vi "Interframe_template-matched-tempbox_displacements_Checked_VI.vi"() -> ()   [LabVIEW 2012]
uses:
  <vilib>/Utility/file.llb/Write To Spreadsheet File (DBL).vi
  <vilib>/imath/engines/lvmath2/RunTimeEngine/NodeEndStatement/NIMS_NodeEndStatement_Output.vi
  <instcachedir>/0/NIMS_NodeEndStatement_Output_53EC0D466D134D7ABD903AC30B43404B.lvgen/NIMS_NodeEndStatement_Output_53EC0D466D134D7ABD903AC30B43404B_001.vi
  <instcachedir>/0/NIMS_NodeEndStatement_Output_53EC0D466D134D7ABD903AC30B43404B.lvgen/NIMS_NodeEndStatement_Output_53EC0D466D134D7ABD903AC30B43404B_005.vi
  <vilib>/imath/engines/lvmath2/RunTimeEngine/ErrorHandling/NIMS_Finalize Error.vi
panel:
  out "Frame\nDelta_X\nDelta_Z":dbl[][](array[numeric])
  out "Matched TempBox (z,x): ROI-Frame_of_Reference":i32[][](array[numeric])
  out "Min_SAD":u32[](array[numeric])
  out "Delta_Z (TempBox-Template)":dbl[](array[numeric])
  out "Delta_X (TempBox-Template)":dbl[](array[numeric])
  in  "ROI in\n2nd frame\n    s_x":dbl=623.0
  in  "ROI in\n2nd frame\n    e_x":dbl=727.0
  in  "ROI in\n2nd frame\n    s_z":dbl=272.0
  in  "ROI in\n2nd frame\n    e_z":dbl=301.0
  out "SAD":u32[][](array[numeric])
  out "SAD_1Darray":u32[](array[numeric])
  out "Frames":T1(plugin-control)
  out "Template in 1st frame of every iteration":u8[][](array[numeric])
  in  "Template \n      in\n1st frame\n     s_x":dbl=658.0
  in  "Template \n      in \n1st frame\n    s_z":dbl=282.0
  in  "Template \n      in \n1st frame\n    e_x":dbl=692.0
  in  "Template \n      in \n1st frame\n    e_z":dbl=291.0
  in  "?":bool
  in  "1st frame":dbl=153.0
  in  "Last frame":dbl=154.0
  out "framesPerSecond":u32
  out "Image Type":T2 items=["Grayscale (U8)", "Grayscale (I16)", "Grayscale (SGL)", "Complex (CSG)", "RGB (U32)", "HSL (U32)", "RGB (U64)"]
  out "Number of Frames":u32
  in  "Path":path=path "C:/Users/admin/Desktop/lohit/pat3.avi"
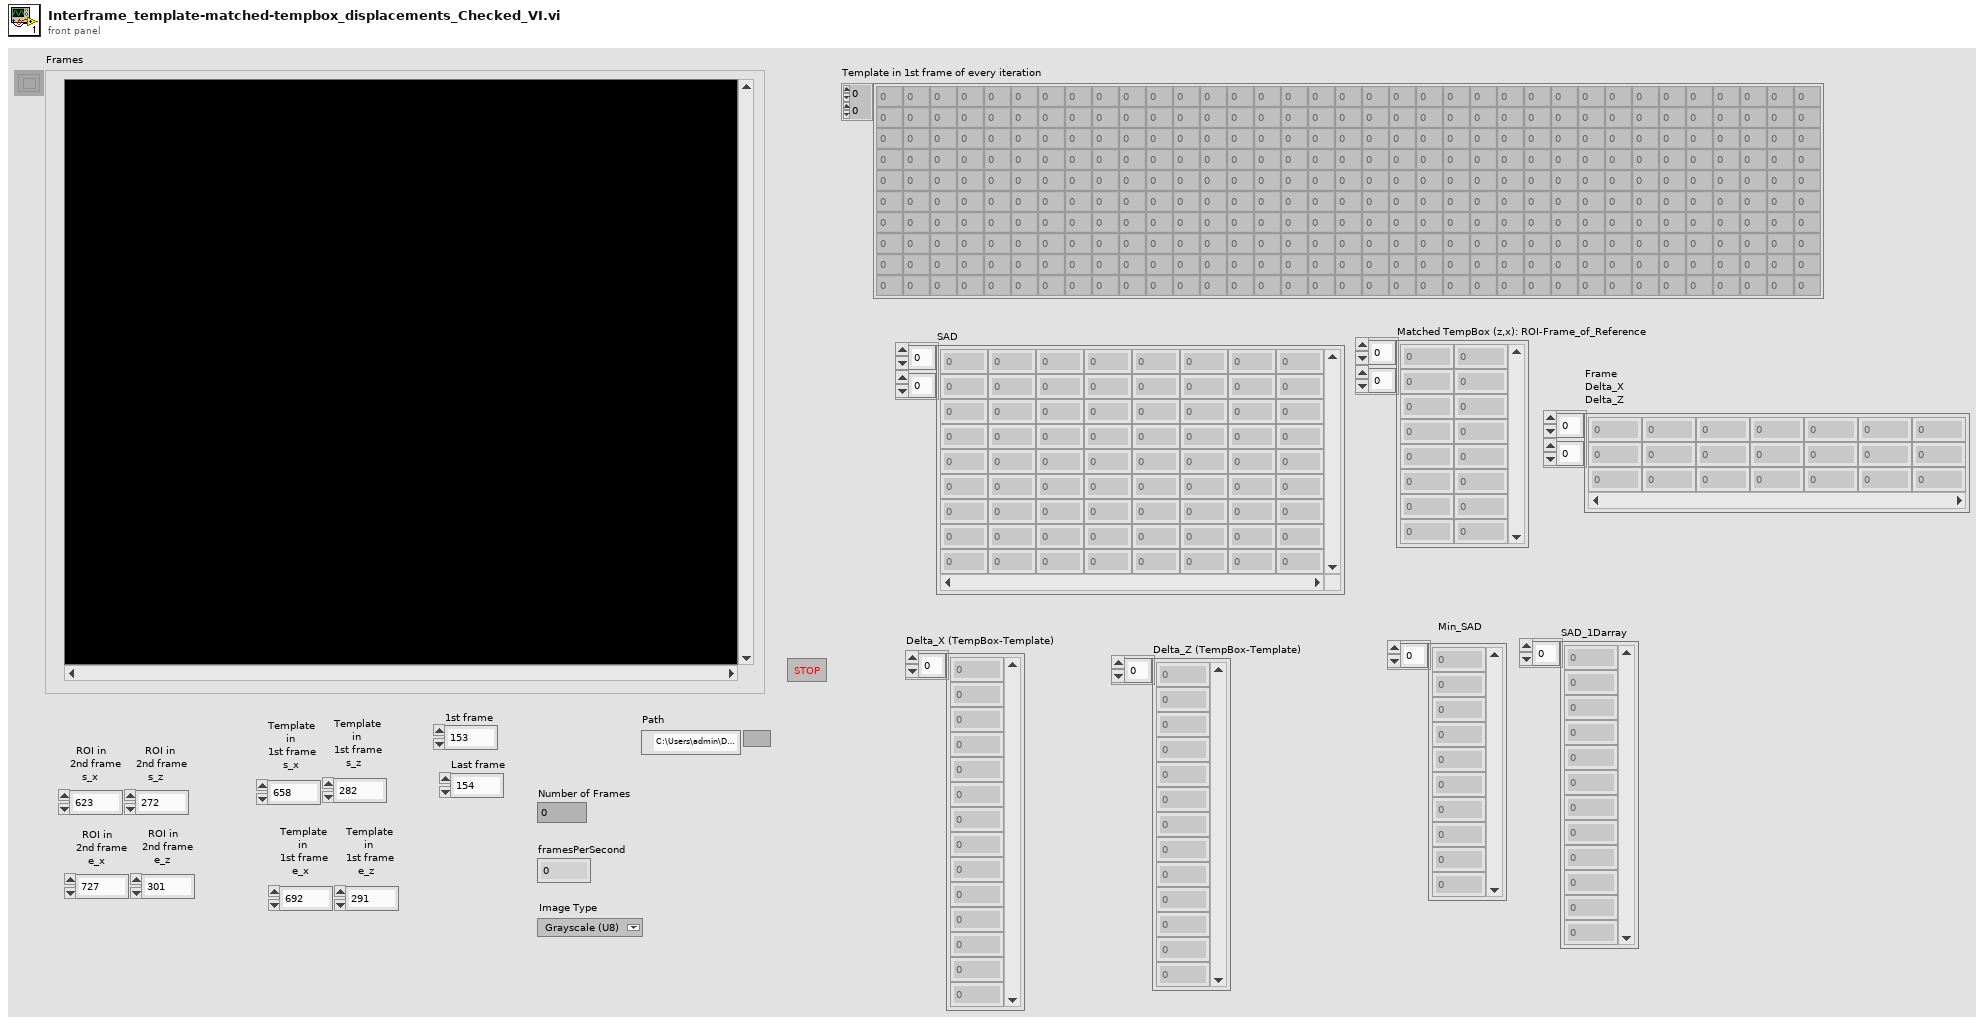
[diagram p1: front panel]
types:
  T1 = typedef "IMAQ Image.ctl" = refnum<image>
  T2 = typedef "Image Type" = u32
  T3 = typedef "AviRefnum.ctl" = refnum<k1>
  T4 = cluster{"width":u32, "height":u32, "framesPerSecond":u32, "compressionFilter":string, "hasData":bool}
  T5 = cluster{"[0]":i32, "[1]":i32, "[2]":i32, "[3]":i32, "[4]":i32, "[5]":i32, "[6]":i32, "[7]":i32, "[8]":i32}
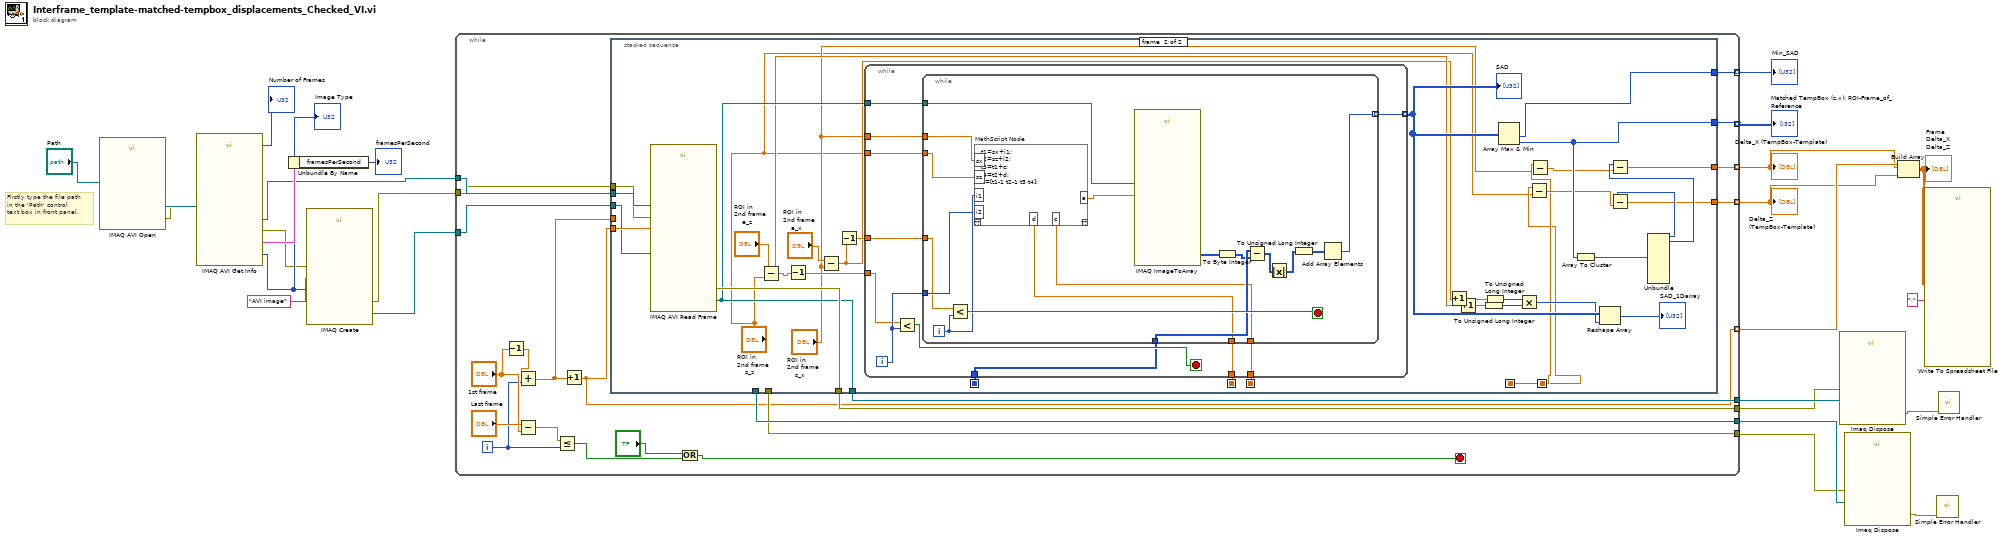
[diagram p0: block diagram]
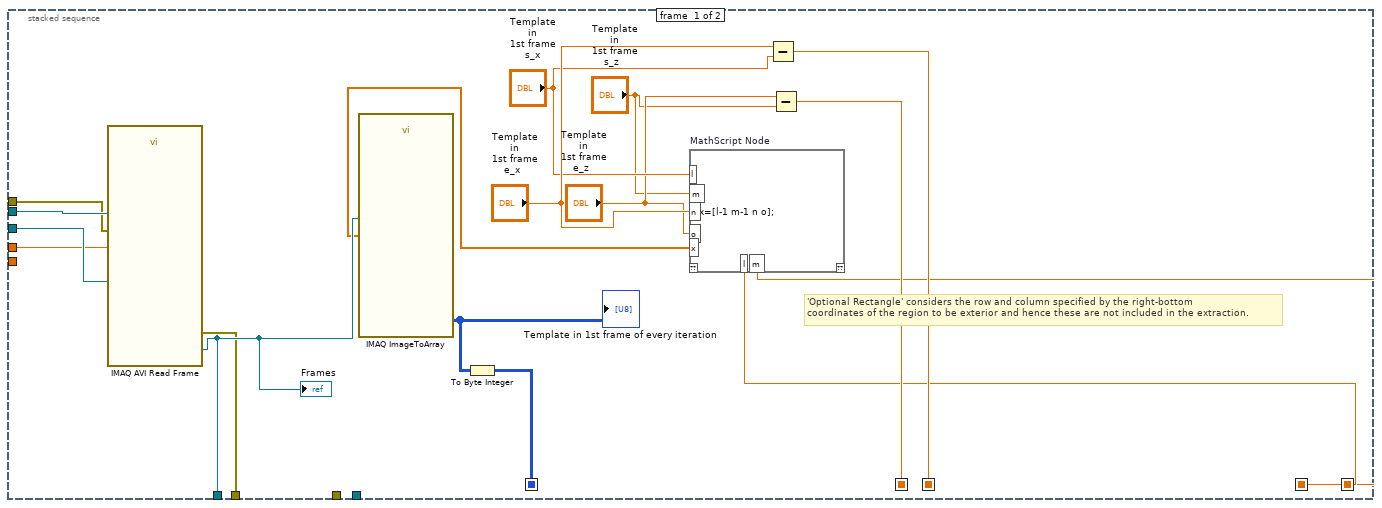
[diagram p2: hidden frame]
diagram:
  # "Firstly type the file path\nin the 'Path' control \ntext box in front panel."
  n1 = call "IMAQ AVI Open"("AVI Path"="Path") -> ("error out"=w18:errorcluster, "Avi Refnum"=w24:T3)  [unwired: 9 in]
  n2 = call "IMAQ AVI Get Info"("error in (no error)"=w18, "Avi Refnum"=w24) -> ("error out"=w17:errorcluster, "Image Type"=w20:T2, "Number of Frames"=→"Number of Frames":u32, "Avi Refnum (duplicate)"=w16:T3, "Frame Data"=w22:T4)  [unwired: 5 in]
  "Image Type" <- w20
  n3 = Unbundle By Name(w22) -> ("framesPerSecond"=→"framesPerSecond":u32)
  n4 = call "IMAQ Create"("Image Name"="AVI image", "Image Type"=w20, "error in (no error)"=w17) -> ("New Image"=w14:T1, "error out"=w15:errorcluster)  [unwired: 2 in]
  n5 = while {
    tunnel: w16 -> [w45]
    tunnel: w15 -> [w44]
    tunnel: w14 -> [w43]
    tunnel: [w40] -> w12
    tunnel: [w39] -> w11
    tunnel: [w38] -> w10
    tunnel: [w37] -> w9
    tunnel: [w36] -> w6 mode=indexing
    tunnel: [w35] -> w5 mode=indexing
    tunnel: [w34] -> w1 mode=indexing
    tunnel: [w31] -> w4 mode=indexing
    tunnel: [w26] -> w7 mode=indexing
    i -> [w28]
    stop <- w46 stop-if-true
    n6 = Decrement(x="1st frame") -> (x-1=w30:dbl)
    n7 = Add(x=w30, y=w28) -> (x+y=w27:dbl)
    n8 = Subtract(x="Last frame", y="1st frame") -> (x-y=w32:dbl)
    n9 = Less Or Equal?(x=w32, y=w28) -> (x <= y?=w42:bool)
    n10 = Increment(x=w27) -> (x+1=w26:dbl)
    n11 = stacked-sequence {
      seq-local: [w59 _] -> [_ w125]
      seq-local: [w51 _] -> [_ w123]
      seq-local: [w52 _] -> [_ w124]
      seq-local: [w50 _] -> [_ w102]
      seq-local: [w49 _] -> [_ w101]
      tunnel: w45 -> [w63 w130]
      tunnel: w44 -> [w62 w128]
      tunnel: w43 -> [w61 w129]
      tunnel: w27 -> [w60 _]
      tunnel: w26 -> [_ w131]
      tunnel: [_ w126] -> w40
      tunnel: [w58 _] -> w39
      tunnel: [w57 _] -> w38
      tunnel: [_ w127] -> w37
      tunnel: [_ w119] -> w36
      tunnel: [_ w118] -> w35
      tunnel: [_ w117] -> w34
      tunnel: [_ w116] -> w31
      frame #0 {
        # "'Optional Rectangle' considers the row and column specified by the right-bottom\ncoordinates of the region to be exterior and hence these are not included in the extraction."
        n12 = call "IMAQ AVI Read Frame"("error in (no error)"=w62, "Frame Number"=w60, "Image"=w61, "Avi Refnum"=w63) -> ("error out"=w57:errorcluster, "Image Out"=w58:T1)  [unwired: 4 in, 2 out]
        "Frames" <- w58
        n13 = mathscript code="x=[l-1 m-1 n o];"("l"="Template \n      in\n1st frame\n     s_x", "m"="Template \n      in \n1st frame\n    s_z", "n"="Template \n      in \n1st frame\n    e_x", "o"="Template \n      in \n1st frame\n    e_z") -> ("x"=w48:dbl[], "l"=w50:dbl, "m"=w49:dbl)  [unwired: 1 in, 1 out]
        n14 = call "IMAQ ImageToArray"("Optional Rectangle"=w48, "Image"=w58) -> ("Image Pixels (U8)"=w47:u8[][])  [unwired: 2 in, 4 out]
        "Template in 1st frame of every iteration" <- w47
        n15 = To Byte Integer(number=w47) -> (8bit integer=w59:i8[][])
        n16 = Subtract(x="Template \n      in \n1st frame\n    e_x", y="Template \n      in\n1st frame\n     s_x") -> (x-y=w52:dbl)
        n17 = Subtract(x="Template \n      in \n1st frame\n    e_z", y="Template \n      in \n1st frame\n    s_z") -> (x-y=w51:dbl)
      }
      frame #1 {
        n18 = call "IMAQ AVI Read Frame"("error in (no error)"=w128, "Frame Number"=w131, "Image"=w129, "Avi Refnum"=w130) -> ("error out"=w127:errorcluster, "Image Out"=w126:T1)  [unwired: 4 in, 2 out]
        n19 = Subtract(x="ROI in\n2nd frame\n    e_z", y="ROI in\n2nd frame\n    s_z") -> (x-y=w108:dbl)
        n20 = Decrement(x=w108) -> (x-1=w109:dbl)
        n21 = Subtract(x="ROI in\n2nd frame\n    e_x", y="ROI in\n2nd frame\n    s_x") -> (x-y=w105:dbl)
        n22 = Decrement(x=w105) -> (x-1=w106:dbl)
        n23 = while {
          tunnel: w126 -> [w141]
          tunnel: w125 -> [w139]
          tunnel: w124 -> [w138]
          tunnel: w123 -> [w137]
          tunnel: [w136] -> w115 mode=indexing
          tunnel: w109 -> [w135]
          tunnel: w106 -> [w134]
          tunnel: "ROI in\n2nd frame\n    s_x" -> [w133]
          tunnel: "ROI in\n2nd frame\n    s_z" -> [w132]
          i -> [w140]
          stop <- w142 stop-if-true
          n24 = Less?(x=w135, y=w140) -> (x < y?=w142:bool)
          n25 = while {
            tunnel: w141 -> [w157]
            tunnel: w140 -> [w155]
            tunnel: w139 -> [w150]
            tunnel: w138 -> [w148]
            tunnel: w137 -> [w147]
            tunnel: [w146] -> w136 mode=indexing
            tunnel: w134 -> [w145]
            tunnel: w133 -> [w144]
            tunnel: w132 -> [w143]
            i -> [w156]
            stop <- w158 stop-if-true
            n26 = Less?(x=w145, y=w156) -> (x < y?=w158:bool)
            n27 = mathscript code="t1=sx+i1;\nt2=sz+i2;\nt3=t1+c;\nt4=t2+d;\na=[t1-1 t2-1 t3 t4];"("sx"=w144, "sz"=w143, "i1"=w156, "i2"=w155, "c"=w148, "d"=w147) -> ("a"=w154:dbl[])  [unwired: 1 in, 1 out]
            n28 = call "IMAQ ImageToArray"("Optional Rectangle"=w154, "Image"=w157) -> ("Image Pixels (U8)"=w159:u8[][])  [unwired: 2 in, 4 out]
            n29 = To Byte Integer(number=w159) -> (8bit integer=w149:i8[][])
            n30 = Subtract(x=w150, y=w149) -> (x-y=w152:i8[][])
            n31 = Absolute Value(x=w152) -> (abs(x)=w151:i8[][])
            n32 = To Unsigned Long Integer(number=w151) -> (unsigned 32bit integer=w153:u32[][])
            n33 = Add Array Elements(numeric array=w153) -> (sum=w146:u32)
          }
        }
        "SAD" <- w115
        n34 = Increment(x=w105) -> (x+1=w98:dbl)
        n35 = Increment(x=w108) -> (x+1=w97:dbl)
        n36 = To Unsigned Long Integer(number=w97) -> (unsigned 32bit integer=w111:u32)
        n37 = To Unsigned Long Integer(number=w98) -> (unsigned 32bit integer=w112:u32)
        n38 = Array Max & Min(array=w115) -> (min value=w117:u32, min index (indices)=w116:i32[])  [unwired: 2 out]
        n39 = Multiply(x=w112, y=w111) -> (x*y=w113:u32)
        n40 = Subtract(x=w101, y="ROI in\n2nd frame\n    s_z") -> (x-y=w104:dbl)
        n41 = Subtract(x=w102, y="ROI in\n2nd frame\n    s_x") -> (x-y=w103:dbl)
        n42 = Array To Cluster(array=w116) -> (cluster=w122:T5)
        n43 = Reshape Array "Reshape Array"(w115, w113) -> (→"SAD_1Darray":u32[])
        n44 = Unbundle "Unbundle"(w122) -> ("[0]"=w120:i32, "[1]"=w121:i32)  [unwired: 7 out]
        n45 = Subtract(x=w121, y=w103) -> (x-y=w119:dbl)
        n46 = Subtract(x=w120, y=w104) -> (x-y=w118:dbl)
      }
    }
    n47 = Or(x="?", y=w42) -> (x .or. y?=w46:bool)
  }
  "Delta_X (TempBox-Template)" <- w6
  "Delta_Z (TempBox-Template)" <- w5
  "Min_SAD" <- w1
  "Matched TempBox (z,x): ROI-Frame_of_Reference" <- w4
  n48 = call "Imaq Dispose"("Image"=w12, "error in (no error)"=w9) -> ("error out"=w13:errorcluster)  [unwired: 4 in]
  n49 = call "Imaq Dispose"("Image"=w11, "error in (no error)"=w10) -> ("error out"=w8:errorcluster)  [unwired: 4 in]
  n50 = Build Array(w7, w6, w5) -> (w3:dbl[][])
  "Frame\nDelta_X\nDelta_Z" <- w3
  n51 = call-poly <vilib>:"Write To Spreadsheet File.vi"("delimiter (\\t)"="," ("delimiter (\\t)"), "2D data"=w3) -> ()  [unwired: 6 in, 1 out]
  n52 = call <vilib>:"Simple Error Handler.vi"("error in (no error)"=w8) -> ()  [unwired: 4 in, 5 out]
  n53 = call <vilib>:"Simple Error Handler.vi"("error in (no error)"=w13) -> ()  [unwired: 4 in, 5 out]
